vi "Manual_stop.vi"(0 "Boolean":bool) -> ()   [LabVIEW 2013]
panel:
  out "Stopped":bool
  out "Moving":bool
  out "Status":string="Initialise"
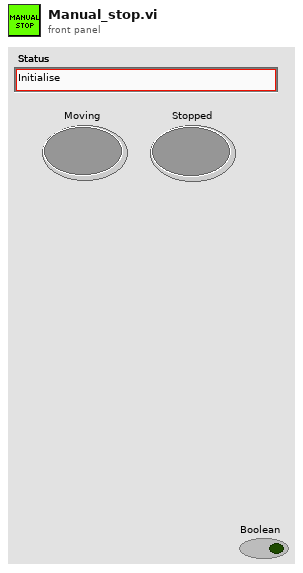
[diagram p1: front panel]
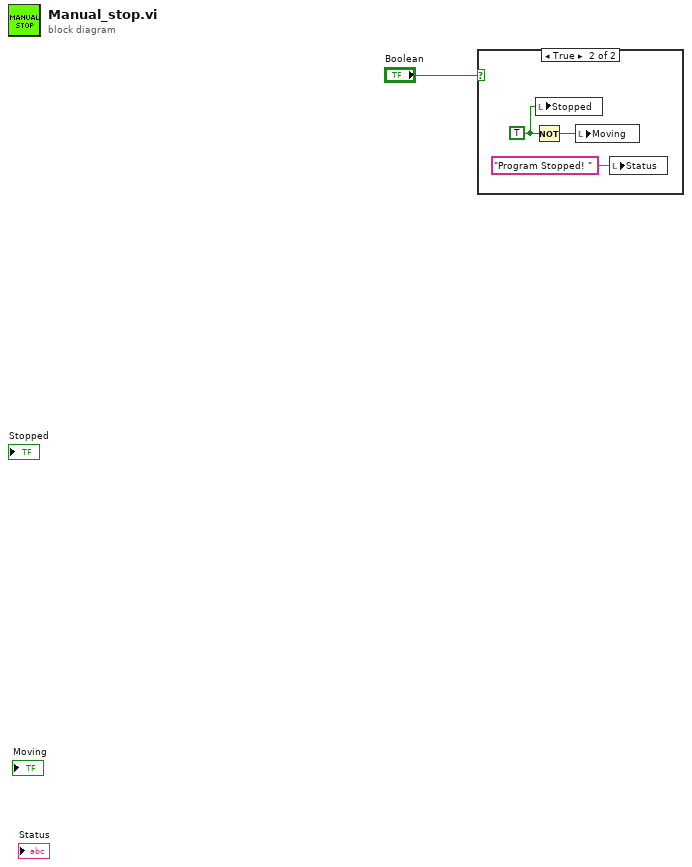
[diagram p0: block diagram]
diagram:
  n1 = case shown="True" "Boolean" {
    frame False {
    }
    frame True {
      w4 = TRUE ("Stopped")
      n2 = Not(x=w4) -> (.not. x?=w3:bool)
      n3 = local write "Stopped"(w4) -> ()
      n4 = local write "Moving"(w3) -> ()
      n5 = local write "Status"("Program Stopped! " ("Status")) -> ()
    }
  }
